vi "Shared Variable Client - Variable Nodes.vi"() -> ()   [LabVIEW 2023]
doc: "This client VI connects to Shared Variable Server.vi by using two Shared Variable nodes on the diagram that are statically linked to the server's shared variables."
panel:
  in  "Stop":bool
  out "Monitor Value 1":dbl(slide) scale=0.0..1.0
  out "Monitor Value 2":dbl(slide) scale=0.0..1.0
  # "Overview: Demonstrates the use of Shared Variable nodes to read shared variable data from a server VI.\nRequirements: Windows\nInstructions:\n1. Make sure Shared Variable Server.vi is already running.\n2. Run this VI. It will read the values of the server's shared variables with Shared Variable nodes.\n3. Click Stop to stop the VI."
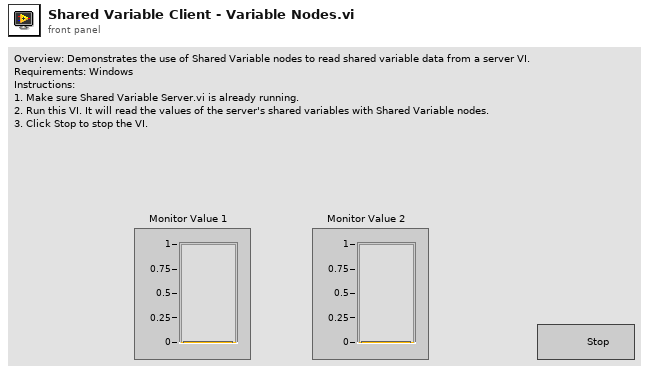
[diagram p1: front panel]
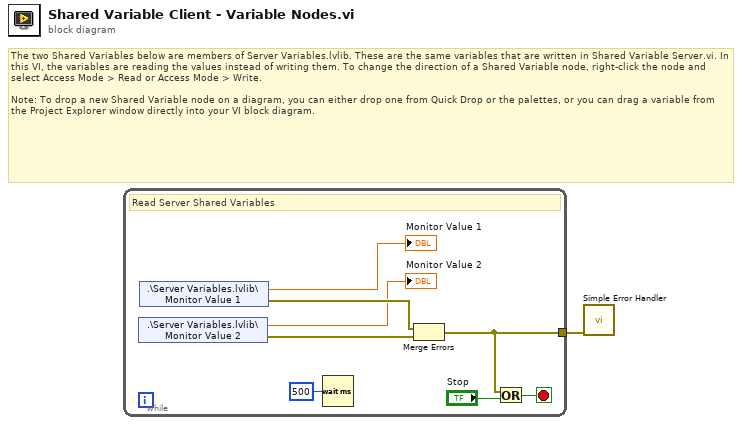
[diagram p0: block diagram]
diagram:
  # "The two Shared Variables below are members of Server Variables.lvlib. These are the same variables that are written in Shared Variable Server.vi. In this VI, the variables are reading the values instead of writing them. To change the direction of a Shared Variable node, right-click the node and select Access Mode > Read or Access Mode > Write.\n\nNote: To drop a new Shared Variable node on a diagram, you can either drop one from Quick Drop or the palettes, or you can drag a variable from the Project Explorer window directly into your VI block diagram."
  n1 = while {
    tunnel: [w4] -> w1
    stop <- w8 stop-if-true
    # "Read Server Shared Variables"
    n2 = shared-variable ".\\Server Variables.lvlib\\Monitor Value 2"() -> (→"Monitor Value 2":dbl, error out=w6:errorcluster)  [unwired: 1 in]
    n3 = shared-variable ".\\Server Variables.lvlib\\Monitor Value 1"() -> (→"Monitor Value 1":dbl, error out=w5:errorcluster)  [unwired: 1 in]
    n4 = Wait (ms)(milliseconds to wait=u32 500 ("millisecond multiple")) -> ()  [unwired: 1 out]
    n5 = Merge Errors(w5, w6) -> (w4:errorcluster)
    n6 = Or(x=w4, y="Stop") -> (x .or. y?=w8:bool)
  }
  n7 = call <vilib>:"Simple Error Handler.vi"("error in (no error)"=w1) -> ()  [unwired: 4 in, 5 out]
